vi "Configure Device.vi"(8 "error in":errorcluster, 11 "Device in":refnum<class "Configurable Device.lvclass">) -> (0 "error out":errorcluster, 3 "Device out":refnum<class "Configurable Device.lvclass">, 4 "SP":dbl, 5 "Settable?":bool)   [LabVIEW 2018, in "Device.lvlib" / "Configurable Device.lvclass"]
doc: "This is the configuration method for the Device object. The one parameter that all should have in common and is not dependent on the configuration of the device is the label which is read from the ini file. All devices that use this class should have this in their configuration."
uses:
  Configurable Device.lvclass
  reusable/Session APIs/File Access/Config Data/Config Data.lvclass
  Configurable Device.lvclass/Configurable Device.ctl
  reusable/Session APIs/File Access/Config Data/Config Data.lvclass/Config Data.ctl
  reusable/Session APIs/File Access/Config Data/Accessors/Read Ref.vi
  <vilib>/Utility/config.llb/Read Key (String).vi
  <vilib>/Utility/config.llb/NI_LVConfig.lvlib
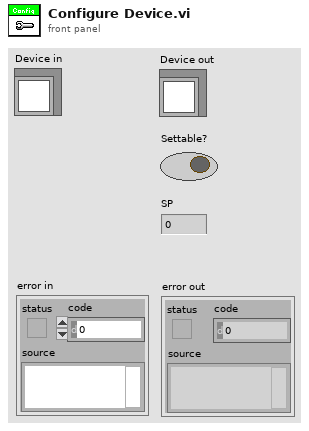
[diagram p1: front panel]
types:
  T1 = typedef "Config Data.lvclass/Config Session.ctl" = refnum<data-value>
  T2 = typedef "NI_LVConfig.lvlib/Config Data RefNum.ctl" = refnum<k1>
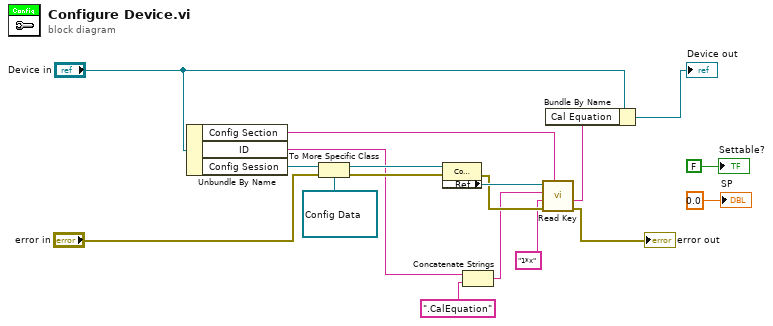
[diagram p0: block diagram]
diagram:
  n1 = Unbundle By Name("Device in") -> ("Config Section"=w1:string, "ID"=w9:string, "Config Session"=w18:T1)
  n2 = To More Specific Class(target class=refnum<data-value> refnum ("Config Session"), reference=w18, error in="error in") -> (specific class reference=w16:refnum<data-value>, error out=w15:errorcluster)
  n3 = property class="Config Data"(reference=w16, error in=w15) -> (error out=w10:errorcluster, "Accessors:Ref"=w11:T2)  [unwired: 1 out]
  n4 = Concatenate Strings(w9, ".CalEquation" ("ID")) -> (w8:string)
  n5 = call-poly <vilib>:"Read Key.vi"("section"=w1, "error in (no error)"=w10, "default value"="1*x", "key"=w8, "refnum"=w11) -> ("error out"=→"error out":errorcluster, "value"=w5:string)  [unwired: 3 in, 2 out]
  n6 = Bundle By Name(cluster="Device in", "Cal Equation"=w5) -> (→"Device out":refnum<class "Configurable Device.lvclass">)
  "SP" <- 0.0 ("SP")
  "Settable?" <- FALSE ("Settable?")
